vi "Change AO Gain (scaled property node) multi board.vi"() -> ()   [LabVIEW 2015]
doc: "I. Description:\nThis example demonstrates how to output a continuous periodic waveform using an internal sample clock.\n\nII. Instructions for Running:\n1. Select the Physical Channel to correspond to where your signal is output on the DAQ device.\n2. Enter the Minimum and Maximum Voltage Ranges\n3. Specify the Desired Frequency of the output Waveform\n4. Enter the Waveform Information. See the documentation of the Waveform Buffer Generation SubVI for information on each parameter.\n\nIII. Block Diagram Steps:\n1. Create an Analog Output Voltage channel.\n2. Call the DAQmx Timing (Use Waveform) VI which sets the sample clock rate based on the input waveform parameters, and set the sample mode to Continuous.\n3. Write the waveform to the output buffer.\n4. Call the Start VI.\n5. Loop continuously until the user presses the Stop button. Check for errors every 100 ms using the Is Task Done? VI\n6. Clear the Task\n7. Use the popup dialog box to display an error or warning if any.\n\nIV. I/O Connections Overview:\nMake sure your signal output terminal matches the Physical Channel I/O Control. For further connection information, refer to your hardware reference manual."
uses:
  <vilib>/DAQmx/create/channels.llb/DAQmx Create Channel (AO-Voltage-Basic).vi
  <vilib>/Utility/error.llb/DialogType.ctl
  <vilib>/DAQmx/configure/timing.llb/DAQmx Timing (Sample Clock).vi
  <vilib>/DAQmx/write.llb/DAQmx Write (Analog 2D DBL NChan NSamp).vi
  <resource>/objmgr/daqmx.rc
panel:
  in  "AO Gain  Property node":dbl(slide) min=-40.0 max=0.0 step=20.0 scale format="%#_2g"
  in  "physical channels 2":tag="PXI1Slot2/ao0" caption="Output Physical Channels"
  out "Resulting Frequency":dbl=1000.0000002037268 format="%.2f"
  in  "Cycles per Buffer":i32=5
  in  "Waveform Type":T1(ring)
  in  "Desired Frequency":dbl=1000.0 format="%.2f"
  in  "Samples per Buffer":dbl=250.0
  in  "Amplitude":dbl=10.0 format="%0.2p"
  out "Waveform Graph":dbl[](graph) caption="Output Waveform"
  in  "Physical Channels":tag="PXI1Slot2/ao0:1"
  in  "Minimum Value":dbl=-10.0 format="%0.2f"
  in  "Maximum Value":dbl=10.0 format="%0.2f"
  in  "stop":bool
  # "Work in progress !"
  # "For instructions, select Help>>Show Context Help"
  # "Channel Parameters"
  # "Timing Parameters"
  # "Waveform Information"
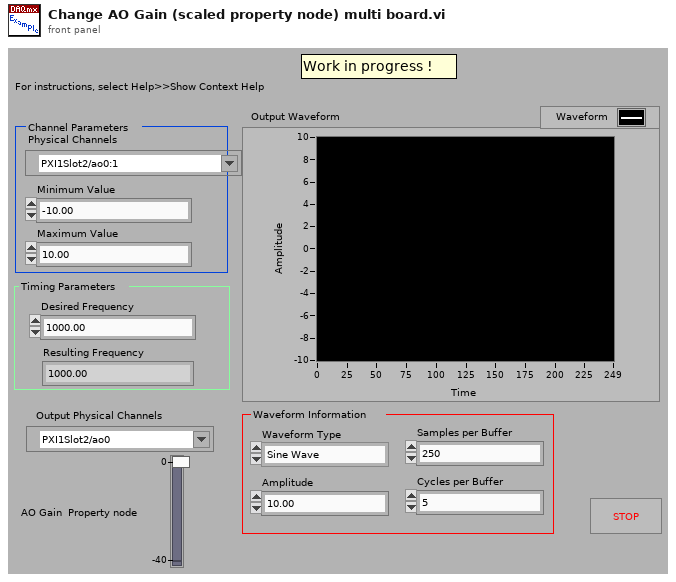
[diagram p1: front panel]
types:
  T1 = enum16{"Sine Wave", "Triangle Wave", "Square Wave", "Sawtooth Wave"}
  T2 = typedef "DialogType.ctl" = u16
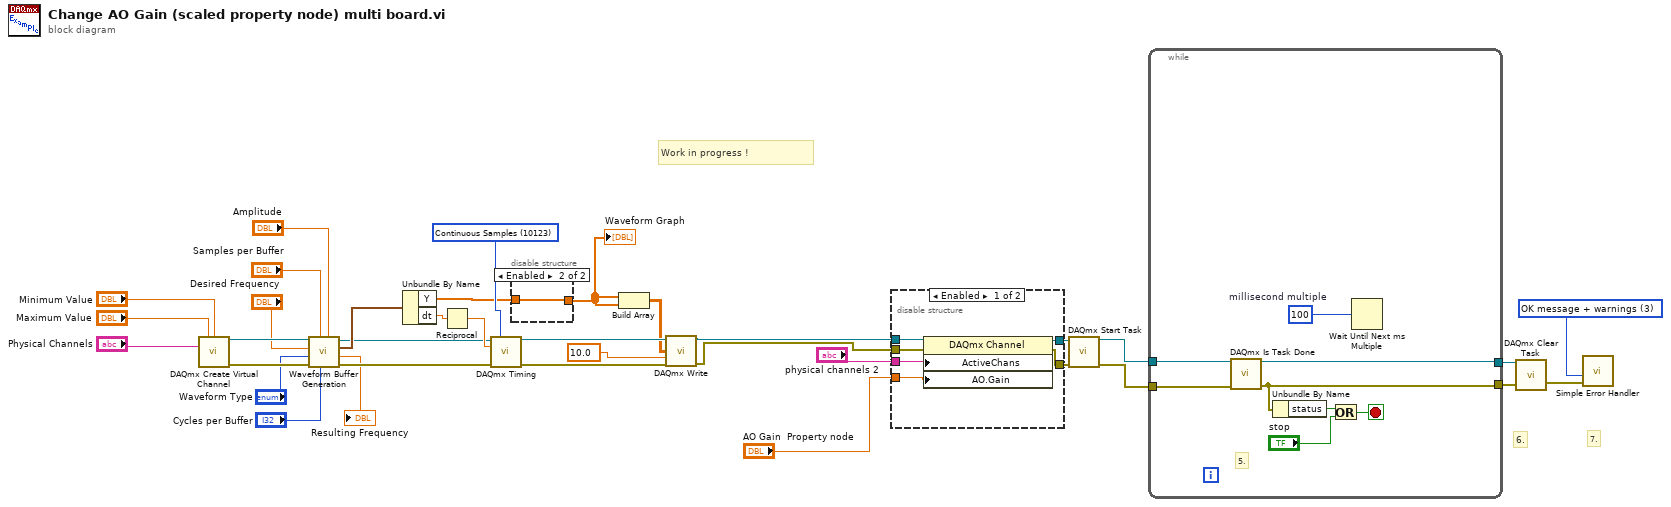
[diagram p0: block diagram]
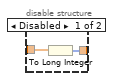
[diagram p2: hidden frame]
diagram:
  w12 = 10123 items=["Finite Samples"=10178, "Continuous Samples"=10123, "Hardware Timed Single Point"=12522] ("sample mode")
  w26 = T2 3 items=["no dialog", "OK message", "continue or stop message", "OK message + warnings", "continue/stop + warnings"] ("type of dialog (OK msg:1)")
  # "Work in progress !"
  # "7."
  # "6."
  n1 = call-poly <vilib>:"DAQmx Create Virtual Channel.vi"("maximum value"="Maximum Value", "minimum value"="Minimum Value", "physical channels"="Physical Channels") -> ("task out"=w22:refnum<k21>, "error out"=w21:errorcluster)  [unwired: 11 in]
  n2 = call "Waveform Buffer Generation.vi"("Amplitude"="Amplitude", "Cycles per Buffer"="Cycles per Buffer", "Samples per Buffer"="Samples per Buffer", "error in (no error)"=w21, "Waveform Type"="Waveform Type", "Desired Frequency"="Desired Frequency", "task/channels in"=w22) -> ("error out"=w23:errorcluster, "Resulting Frequency"=→"Resulting Frequency":dbl, "Waveform"=w15:waveform(dbl), "task out"=w9:refnum<k21>)  [unwired: 1 out]
  n3 = Unbundle By Name(w15) -> ("Y"=w2:dbl[], "dt"=w14:dbl)
  n4 = Reciprocal(x=w14) -> (1/x=w13:dbl)
  n5 = call-poly <vilib>:"DAQmx Timing.vi"("task/channels in"=w9, "sample mode"=w12, "rate"=w13, "error in"=w23) -> ("task out"=w29:refnum<k21>, "error out"=w28:errorcluster)  [unwired: 10 in]
  n6 = disable-structure shown="Enabled" {
    disable-tunnel: [w37 w38] -> w3
    disable-tunnel: w2 -> [w36 w38]
    frame Disabled {
      n7 = To Long Integer(number=w36) -> (32bit integer=w37:i32[])
    }
    frame Enabled {
    }
  }
  "Waveform Graph" <- w3
  n8 = Build Array(w3, w3) -> (w11:dbl[][])
  n9 = call-poly <vilib>:"DAQmx Write.vi"("task/channels in"=w29, "data"=w11, "timeout"=10.0 ("Wirite Timeout"), "error in"=w28) -> ("task out"=w7:refnum<k21>, "error out"=w4:errorcluster)  [unwired: 9 in, 1 out]
  n10 = disable-structure shown="Enabled" {
    disable-tunnel: "AO Gain  Property node" -> [w44 _]
    disable-tunnel: "physical channels 2" -> [w43 _]
    disable-tunnel: w7 -> [w42 w46]
    disable-tunnel: [w41 w46] -> w6
    disable-tunnel: [w40 w45] -> w5
    disable-tunnel: w4 -> [w39 w45]
    frame Enabled {
      n11 = property class="DAQmx Channel"(reference=w42, error in=w39, "ActiveChans"=w43, "AO.Gain"=w44) -> (reference out=w41:refnum<k21>, error out=w40:errorcluster)
    }
    frame Disabled {
    }
  }
  n12 = call <vilib>:"DAQmx Start Task.vi"("task/channels in"=w6, "error in"=w5) -> ("task out"=w27:refnum<k21>, "error out"=w31:errorcluster)  [unwired: 12 in]
  n13 = while {
    tunnel: w27 -> [w54]
    tunnel: [w53] -> w25
    tunnel: w31 -> [w52]
    tunnel: [w51] -> w24
    stop <- w49 stop-if-true
    w50 = u32 100  # millisecond multiple
    # "5."
    n14 = call <vilib>:"DAQmx Is Task Done.vi"("task/channels in"=w54, "error in"=w52) -> ("task out"=w53:refnum<k21>, "error out"=w51:errorcluster)  [unwired: 11 in, 1 out]
    n15 = Unbundle By Name(w51) -> ("status"=w48:bool)
    n16 = Or(x=w48, y="stop") -> (x .or. y?=w49:bool)
    n17 = Wait Until Next ms Multiple(millisecond multiple=w50) -> ()  [unwired: 1 out]
  }
  n18 = call <vilib>:"DAQmx Clear Task.vi"("task in"=w25, "error in"=w24) -> ("error out"=w35:errorcluster)  [unwired: 13 in]
  n19 = call <vilib>:"Simple Error Handler.vi"("type of dialog (OK msg:1)"=w26, "error in (no error)"=w35) -> ()  [unwired: 3 in, 5 out]
